vi "Convert_measure_line.vi"(11 "sequence line":string[](array[string])) -> (3 "command":string[](array[string]))   [LabVIEW 2017]
panel:
  out "文字列":string
  in  "ダミー":string[](array[string])
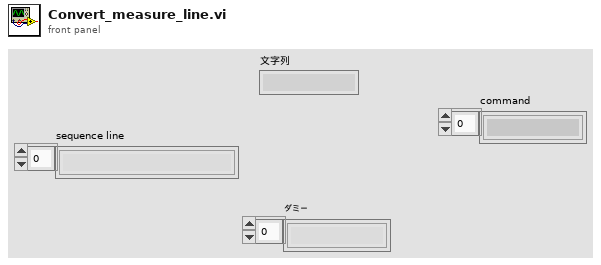
[diagram p1: front panel]
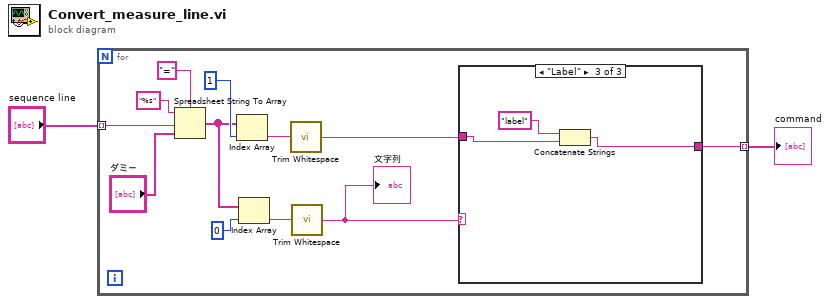
[diagram p0: block diagram]
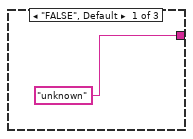
[diagram p2: hidden frame]
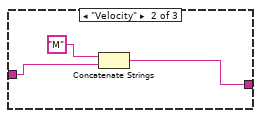
[diagram p3: hidden frame]
diagram:
  n1 = for {
    tunnel: "sequence line" -> [w14] mode=indexing
    tunnel: [w7] -> w1 mode=indexing
    n2 = Spreadsheet String To Array(delimiter (Tab)="=", format string="%s", spreadsheet string=w14, array type (2D Dbl)="ダミー") -> (array=w9:string[])
    n3 = Index Array(array=w9, index=1) -> (element=w5:string)
    n4 = Index Array(array=w9, index=0) -> (element=w6:string)
    n5 = call <vilib>:"Trim Whitespace.vi"("string"=w5) -> ("trimmed string"=w4:string)  [unwired: 1 in]
    n6 = call <vilib>:"Trim Whitespace.vi"("string"=w6) -> ("trimmed string"=w3:string)  [unwired: 1 in]
    "文字列" <- w3
    n7 = case shown="\"Label\"" w3 {
      tunnel: w4 -> [_ w17 w21]
      tunnel: ["unknown" w16 w19] -> w7
      frame "FALSE", Default {
      }
      frame "Velocity" {
        n8 = Concatenate Strings("M", w17) -> (w16:string)
      }
      frame "Label" {
        n9 = Concatenate Strings("label", w21) -> (w19:string)
      }
    }
  }
  "command" <- w1
